vi "number1_sub1-data acquisition.vi"(4 "#s":dbl=10000.0 format="%0.2p", 5 "Fs":dbl=1000.0 format="%0.2p") -> (1 "Waveform Graph":waveform(dbl)(graph))   [LabVIEW 2014]
uses:
  <vilib>/measure/NI_MABase.lvlib
panel:
  in  "OK Button":bool
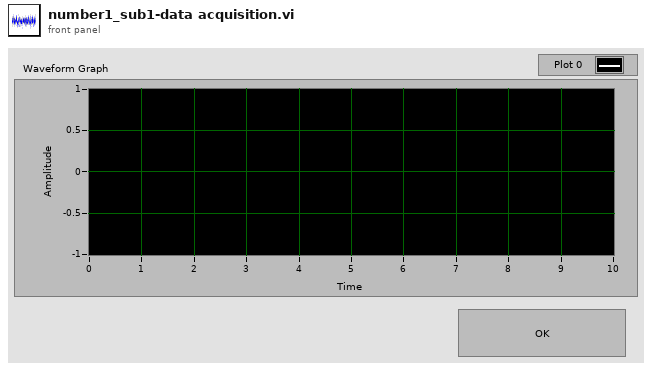
[diagram p1: front panel]
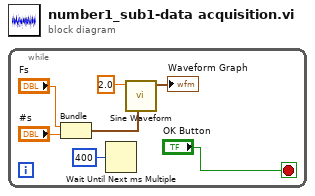
[diagram p0: block diagram]
diagram:
  n1 = while {
    stop <- "OK Button" stop-if-true
    n2 = Bundle("Fs"="Fs", "#s"="#s") -> (w6:cluster{"Fs":dbl, "#s":dbl})  [unwired: 1 in]
    n3 = Wait Until Next ms Multiple(millisecond multiple=u32 400) -> ()  [unwired: 1 out]
    n4 = call <vilib>:"Sine Waveform.vi"("sampling info"=w6, "frequency"=2.0) -> ("signal out"=→"Waveform Graph":waveform(dbl))  [unwired: 8 in, 1 out]
  }
